vi "题目5.vi"() -> ()   [LabVIEW 2017]
panel:
  in  "可见":bool
  in  "停止":bool
  out "波形图":dbl[](graph)
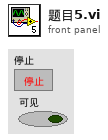
[diagram p1: front panel]
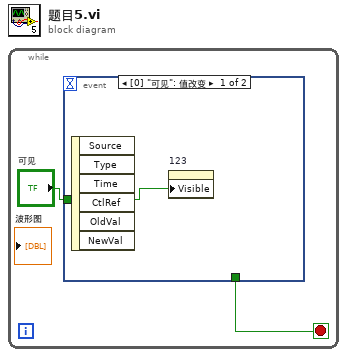
[diagram p0: block diagram]
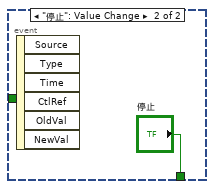
[diagram p2: hidden frame]
diagram:
  n1 = while {
    stop <- w1 stop-if-true
    n2 = event shown="[0] \"可见\": 值改变" {
      selector: _ -> [_ _]
      dyn-events: _ -> [_ _]
      timeout: _ -> [_ _]
      tunnel: "可见" -> [w3 _]
      tunnel: [_ "停止"] -> w1
      event "可见": Value Change {
        n3 = event-data() -> ()  [unwired: 1 in, 6 out]
        n4 = property on="123" class="WFGraph (严格)"("Visible"=w3) -> ()  [unwired: 2 in, 2 out]
      }
      event "停止": Value Change {
        n5 = event-data() -> ()  [unwired: 1 in, 6 out]
      }
    }
  }
